vi "Wave Gen.vi"() -> ()   [LabVIEW 2018]
panel:
  in  "Filename":string
  in  "File Directory":path
  out "Output Directory":path
  in  "format string":string
  out "error out 2":errorcluster
  out "Output Filename":path
  out "error out":errorcluster
  out "VISA resource name out":refnum<visa-resource-name>
  in  "True To \ngenerate\n pulse":bool
  in  "Rise (20 ns)":dbl=2e-08 format="%#.3g"
  in  "Delay (0.00 s)":dbl min=-1000000.0 max=1000000.0
  in  "Duty (20%)":dbl=20.0 min=0.0001 max=100.0 format="%.4g"
  in  "Fall (20 ns)":dbl=2e-08 format="%#.3g"
  in  "Phase (0.0 degrees)":dbl=0.002 min=-360.0 max=360.0 format="%#.1g"
  in  "Waveform Function (0: Sine) in":u16(ring) items=["Sine", "Square", "Ramp", "DC", "Pulse", "Arb"]
  in  "DC Offset (0.00 V) in":dbl
  in  "Frequency (1000 Hz)":dbl=1000.0 format="%#.6g"
  in  "Amplitude (1.0 Vpp)":dbl=1.0 format="%#.3f"
  in  "Enable Output (T: Enable)":bool=TRUE
  in  "Channel (1:Channel 1)":i32(ring)=1 items=["Channel 1"=1, "Channel 2"=2]
  in  "VISA Refnum in":refnum<visa-resource-name>
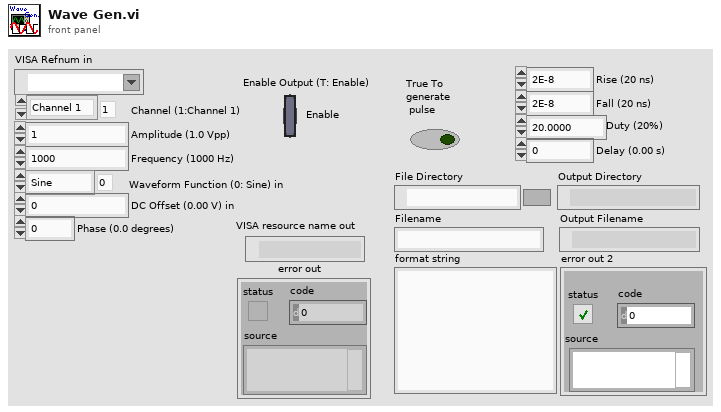
[diagram p1: front panel]
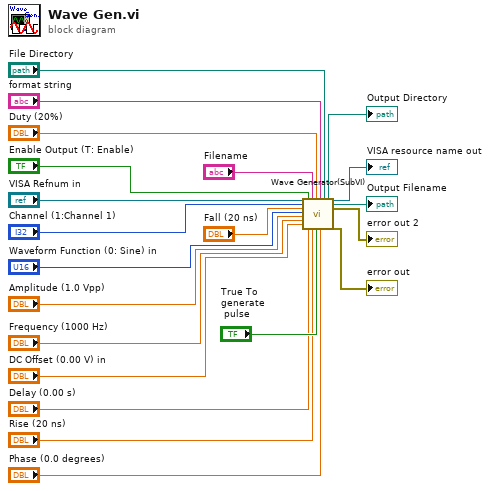
[diagram p0: block diagram]
diagram:
  n1 = call "Wave Generator(SubVI).vi"("VISA Refnum in"="VISA Refnum in", "Channel (1:Channel 1)"="Channel (1:Channel 1)", "Fall (20 ns)"="Fall (20 ns)", "Waveform Function (0: Sine) in"="Waveform Function (0: Sine) in", "Amplitude (1.0 Vpp)"="Amplitude (1.0 Vpp)", "Frequency (1000 Hz)"="Frequency (1000 Hz)", "DC Offset (0.00 V) in"="DC Offset (0.00 V) in", "Enable Output (T: Enable)"="Enable Output (T: Enable)", "Delay (0.00 s)"="Delay (0.00 s)", "Filename"="Filename", "Rise (20 ns)"="Rise (20 ns)", "Duty (20%)"="Duty (20%)", "True To \ngenerate\n pulse"="True To \ngenerate\n pulse", "format string"="format string", "Phase (0.0 degrees)"="Phase (0.0 degrees)", "File Directory"="File Directory") -> ("Output Directory"=→"Output Directory":path, "VISA Refnum out"=→"VISA resource name out":refnum<visa-resource-name>, "Output Filename"=→"Output Filename":path, "error out 2"=→"error out 2":errorcluster, "error out"=→"error out":errorcluster)  [unwired: 7 in]
